vi "Configure Terminals.vi"(11 "State in":T2) -> (2 "cancelled?":bool, 3 "State out":T2)   [LabVIEW 2015, in "LVJSON.lvlib" / "Shared.lvlib"]
uses:
  Shared.lvlib
  Get Object Parameters/State.ctl
  Get Object Parameters/Parameter.ctl
  Get Object Parameters/Get Object Parameters.xnode
panel:
  in  "Terminals":T1[](array[typedef])
  in  "Cancel_Button":bool
  in  "OK_Button":bool
  # "Parameter Name"
  # "JSON Type"
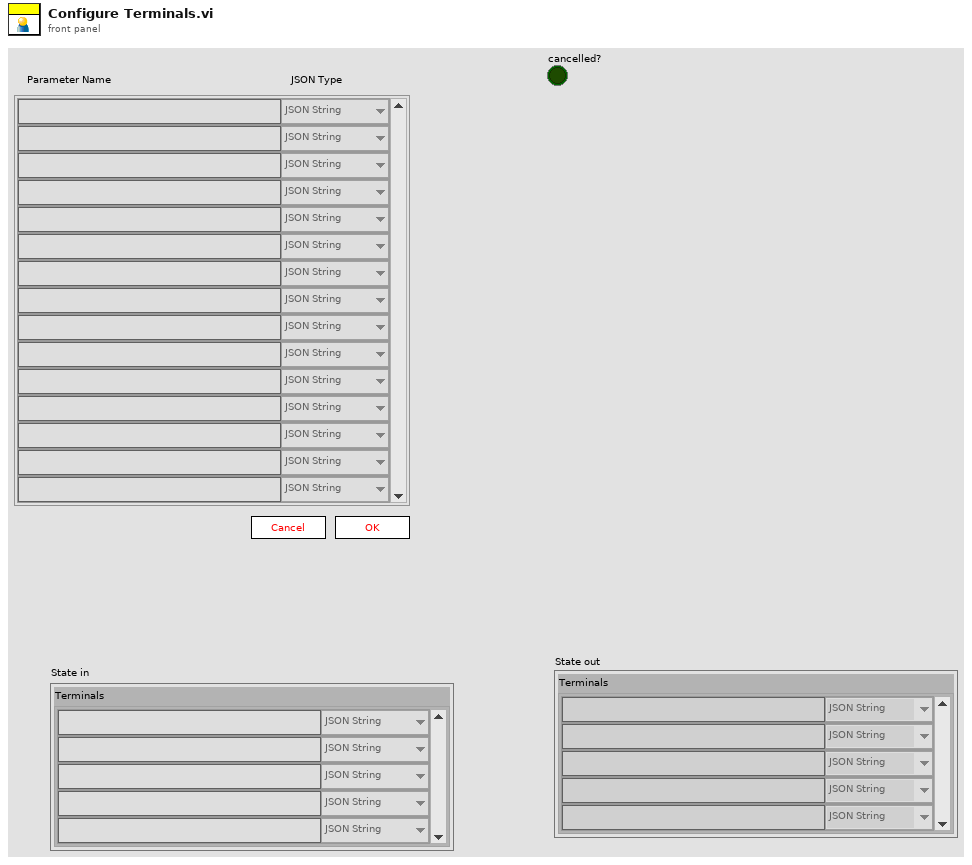
[diagram p1: front panel]
types:
  T1 = typedef "LVJSON.lvlib/Shared.lvlib/Parameter.ctl" = cluster{"Parameter Name":string, "JSON Type":enum16{"JSON String", "JSON Numeric", "JSON Boolean", "JSON", "JSON Object", "JSON Array", "String Value", "Numeric Value", "Boolean Value"}}
  T2 = typedef "LVJSON.lvlib/Get Object Parameters.xnode/State.ctl" = cluster{"Terminals":T1[]}
  T3 = typedef "eventvkey.ctl" = enum16{"ASCII", "Enter", "Return", "Shift", "Ctrl", "Alt", "Cmd", "Opt", "Caps", "NumLock", "Clear", "Break", "Up", "Down", "Left", "Right", "Insert", "Delete", "Home", "End", "PageUp", "PageDown", "Escape", "Help", "Pause", "ScrollLock", "F1", "F2", "F3", "F4", "F5", "F6", "F7", "F8", "F9", "F10", "F11", "F12", "F13", "F14", "F15", "F16", "F17", "F18", "F19", "F20", "F21", "F22", "F23", "F24", "Play", "VolumeUp", "VolumeDown", "Mute", "Two Byte Char"}
  T4 = cluster{"Shift":bool, "Ctrl":bool, "Alt":bool, "Cmd":bool, "Opt":bool}
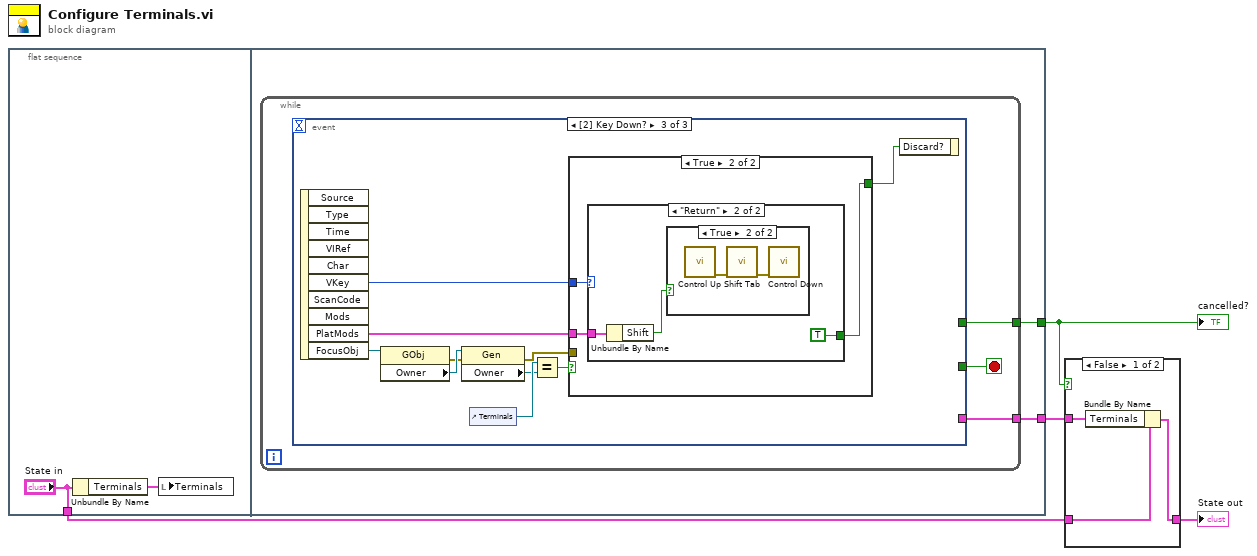
[diagram p0: block diagram]
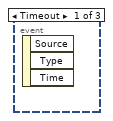
[diagram p3: hidden frame]
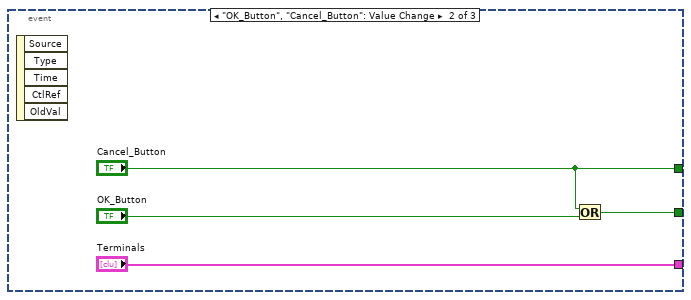
[diagram p4: hidden frame]
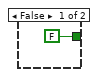
[diagram p5: hidden frame]
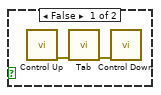
[diagram p7: hidden frame]
diagram:
  n1 = flat-sequence {
    tunnel: ["State in"] -> w4
    tunnel: [w7] -> w2
    tunnel: [w8] -> w1
    frame #0 {
      n2 = Unbundle By Name("State in") -> ("Terminals"=w5:T1[])
      n3 = local write "Terminals"(w5) -> ()
    }
    frame #1 {
      n4 = while {
        tunnel: [w11] -> w8
        tunnel: [w9] -> w7
        stop <- w10 stop-if-true
        n5 = event shown="[2] Key Down?" {
          selector: _ -> [_ _ _]
          dyn-events: _ -> [_ _ _]
          timeout: _ -> [_ _ _]
          tunnel: [_ "Cancel_Button" _] -> w11
          tunnel: [_ w13 _] -> w10
          tunnel: [_ "Terminals" _] -> w9
          event Timeout {
            n6 = event-data() -> ()  [unwired: 1 in, 3 out]
          }
          event "OK_Button", "Cancel_Button": Value Change {
            n7 = event-data() -> ()  [unwired: 1 in, 5 out]
            n8 = Or(x="Cancel_Button", y="OK_Button") -> (x .or. y?=w13:bool)
          }
          event Key Down? {
            n9 = event-data() -> ("VKey"=w25:T3, "PlatMods"=w23:T4, "FocusObj"=w22:refnum<vi>)  [unwired: 1 in, 7 out]
            n10 = property class="GObj"(reference=w22) -> (error out=w17:errorcluster, "Owner"=w19:refnum<vi>)  [unwired: 1 in, 1 out]
            n11 = property class="Gen"(reference=w19, error in=w17) -> (error out=w16:errorcluster, "Owner"=w18:refnum<vi>)  [unwired: 1 out]
            n12 = control-ref of="Terminals"() -> (w21:refnum<vi>)
            n13 = Equal?(x=w21, y=w18) -> (x = y?=w20:bool)
            n14 = case shown="True" w20 {
              tunnel: w25 -> [_ w29]
              tunnel: [FALSE ("Discard?") w28] -> w24
              tunnel: w23 -> [_ w27]
              tunnel: w16 -> [_ _]
              frame False {
              }
              frame True {
                n15 = case shown="\"Return\"" w29 {
                  tunnel: [_ TRUE ("Discard?")] -> w28
                  tunnel: w27 -> [_ w31]
                  frame "ASCII", Default {
                  }
                  frame "Return" {
                    n16 = Unbundle By Name(w31) -> ("Shift"=w30:bool)
                    n17 = case shown="True" w30 {
                      frame False {
                        n18 = call "Control Up.vi"() -> ("error out"=w34:errorcluster)  [unwired: 11 in]
                        n19 = call "Tab.vi"("error in (no error)"=w34) -> ("error out"=w33:errorcluster)  [unwired: 10 in]
                        n20 = call "Control Down.vi"("error in (no error)"=w33) -> ()  [unwired: 10 in, 1 out]
                      }
                      frame True {
                        n21 = call "Control Up.vi"() -> ("error out"=w36:errorcluster)  [unwired: 11 in]
                        n22 = call "Shift Tab.vi"("error in (no error)"=w36) -> ("error out"=w35:errorcluster)  [unwired: 10 in]
                        n23 = call "Control Down.vi"("error in (no error)"=w35) -> ()  [unwired: 10 in, 1 out]
                      }
                    }
                  }
                }
              }
            }
            n24 = event-data("Discard?"=w24) -> ()  [unwired: 1 in, 1 out]
          }
        }
      }
    }
  }
  n25 = case shown="False" w1 {
    tunnel: w4 -> [w39 w40]
    tunnel: [w38 w40] -> w3
    tunnel: w2 -> [w37 _]
    frame False {
      n26 = Bundle By Name(cluster=w39, "Terminals"=w37) -> (w38:T2)
    }
    frame True {
    }
  }
  "State out" <- w3
  "cancelled?" <- w1
